vi "SpringDamperForceGR_virtualWall.vi"(1 "MotorVelocity":dbl, 2 "MotorPosition":dbl, 3 "ForceFromOtherComponents":dbl, 4 "SpringDampers":T1(array[cluster])) -> (0 "Force":dbl)   [LabVIEW 2019]
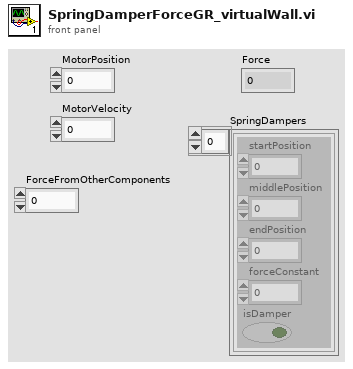
[diagram p1: front panel]
types:
  T1 = cluster{"startPosition":dbl, "middlePosition":dbl, "endPosition":dbl, "forceConstant":dbl, "isDamper":bool}[]
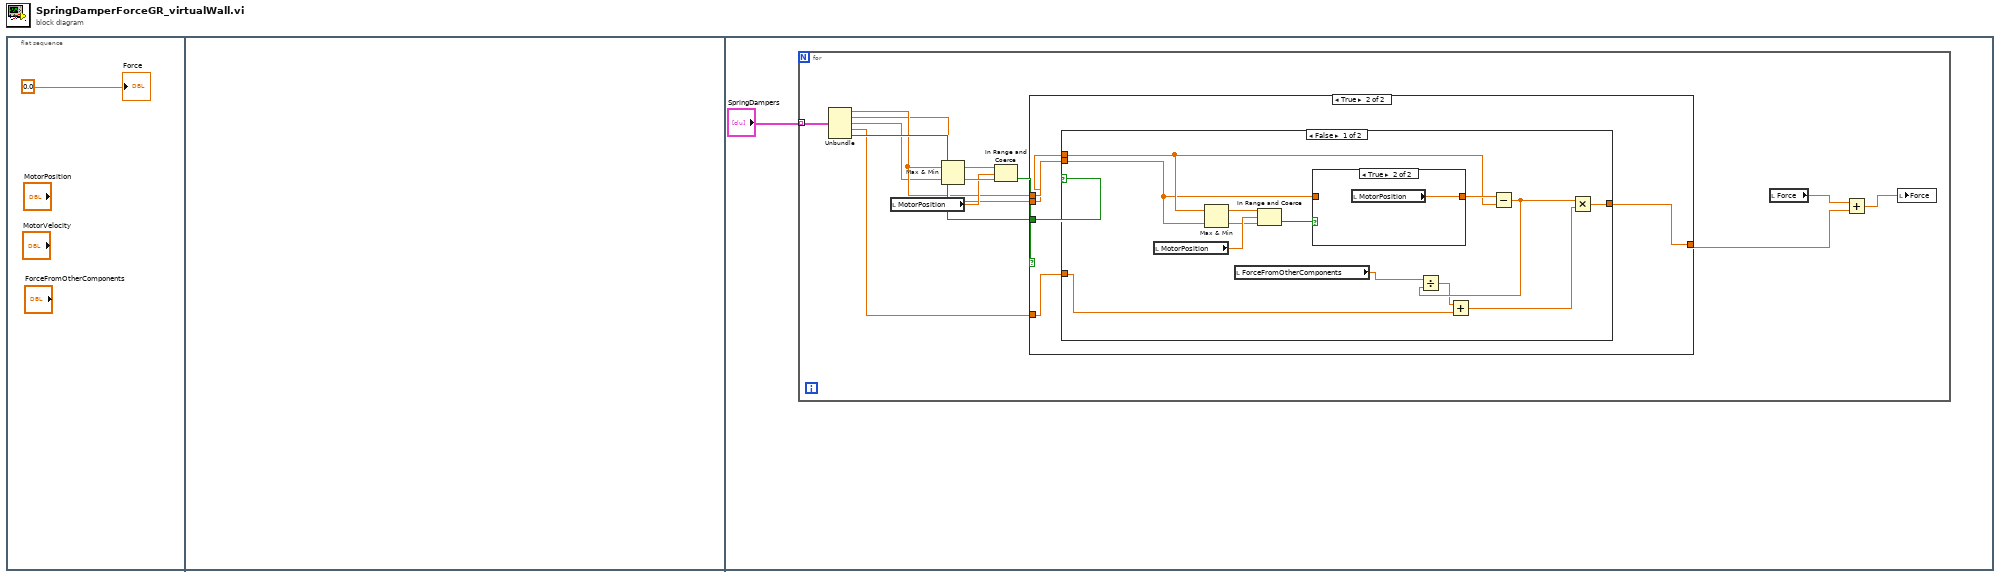
[diagram p0: block diagram]
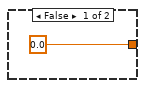
[diagram p2: hidden frame]
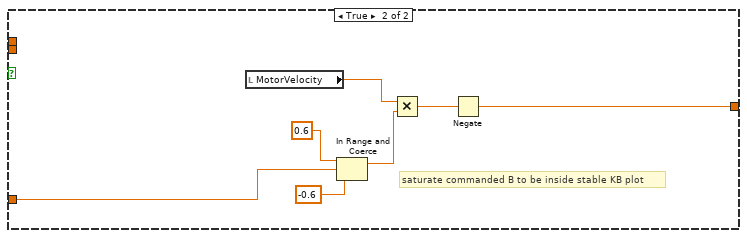
[diagram p4: hidden frame]
diagram:
  n1 = flat-sequence {
    frame #0 {
      "Force" <- 0.0
    }
    frame #1 {
    }
    frame #2 {
      n2 = for {
        tunnel: "SpringDampers" -> [w15] mode=indexing
        n3 = Unbundle(w15) -> ("startPosition"=w5:dbl, "middlePosition"=w3:dbl, "endPosition"=w4:dbl, "forceConstant"=w6:dbl, "isDamper"=w14:bool)
        n4 = local read "MotorPosition"() -> (w8:dbl)
        n5 = Max & Min(x=w5, y=w4) -> (max(x,y)=w9:dbl, min(x,y)=w10:dbl)
        n6 = In Range and Coerce(upper limit=w9, x=w8, lower limit=w10) -> (In Range?=w11:bool)  [unwired: 1 out]
        n7 = case shown="True" w11 {
          tunnel: w14 -> [_ w21]
          tunnel: [0.0 w19] -> w7
          tunnel: w6 -> [_ w20]
          tunnel: w5 -> [_ w18]
          tunnel: w3 -> [_ w17]
          frame False {
          }
          frame True {
            n8 = case shown="False" w21 {
              tunnel: w20 -> [w23 w37]
              tunnel: [w28 w41] -> w19
              tunnel: w18 -> [w29 _]
              tunnel: w17 -> [w27 _]
              frame False {
                n9 = local read "MotorPosition"() -> (w34:dbl)
                n10 = Max & Min(x=w29, y=w27) -> (max(x,y)=w33:dbl, min(x,y)=w32:dbl)
                n11 = local read "ForceFromOtherComponents"() -> (w26:dbl)
                n12 = In Range and Coerce(upper limit=w33, x=w34, lower limit=w32) -> (In Range?=w31:bool)  [unwired: 1 out]
                n13 = case shown="True" w31 {
                  tunnel: [w35 w36] -> w30
                  tunnel: w27 -> [w35 _]
                  frame False {
                  }
                  frame True {
                    n14 = local read "MotorPosition"() -> (w36:dbl)
                  }
                }
                n15 = Subtract(x=w30, y=w29) -> (x-y=w25:dbl)
                n16 = Divide(x=w26, y=w25) -> (x/y=w24:dbl)
                n17 = Add(x=w24, y=w23) -> (x+y=w22:dbl)
                n18 = Multiply(x=w25, y=w22) -> (x*y=w28:dbl)
              }
              frame True {
                # "saturate commanded B to be inside stable KB plot"
                n19 = local read "MotorVelocity"() -> (w43:dbl)
                n20 = In Range and Coerce(upper limit=0.6, x=w37, lower limit=-0.6) -> (coerced(x)=w38:dbl)  [unwired: 1 out]
                n21 = Multiply(x=w43, y=w38) -> (x*y=w42:dbl)
                n22 = Negate(x=w42) -> (-x=w41:dbl)
              }
            }
          }
        }
        n23 = local read "Force"() -> (w13:dbl)
        n24 = Add(x=w13, y=w7) -> (x+y=w12:dbl)
        n25 = local write "Force"(w12) -> ()
      }
    }
  }
